vi "Remove Comments.vi"(8 "error in (no error)":errorcluster, 11 "input string":string="{\n\"Cluster\": {\n\"Name\": \"test\", //Represents the name of a person\n\"Department\": \"test2\"/*Gives the department name and \nthe functionality of the department*/\n}") -> (0 "error out":errorcluster, 3 "output String":string)   [LabVIEW 2015]
doc: "This VI removes comments from the JSON that has just been read from a JSON file.This step is mandatory before parsing out the data to the next step. \nIt is capable of removing <b>single line ( // // ) </b>and<b> multiple line (/* */)</b>comments from the input JSON String."
panel:
  # "The input can be changed to test the working of the SubVI"
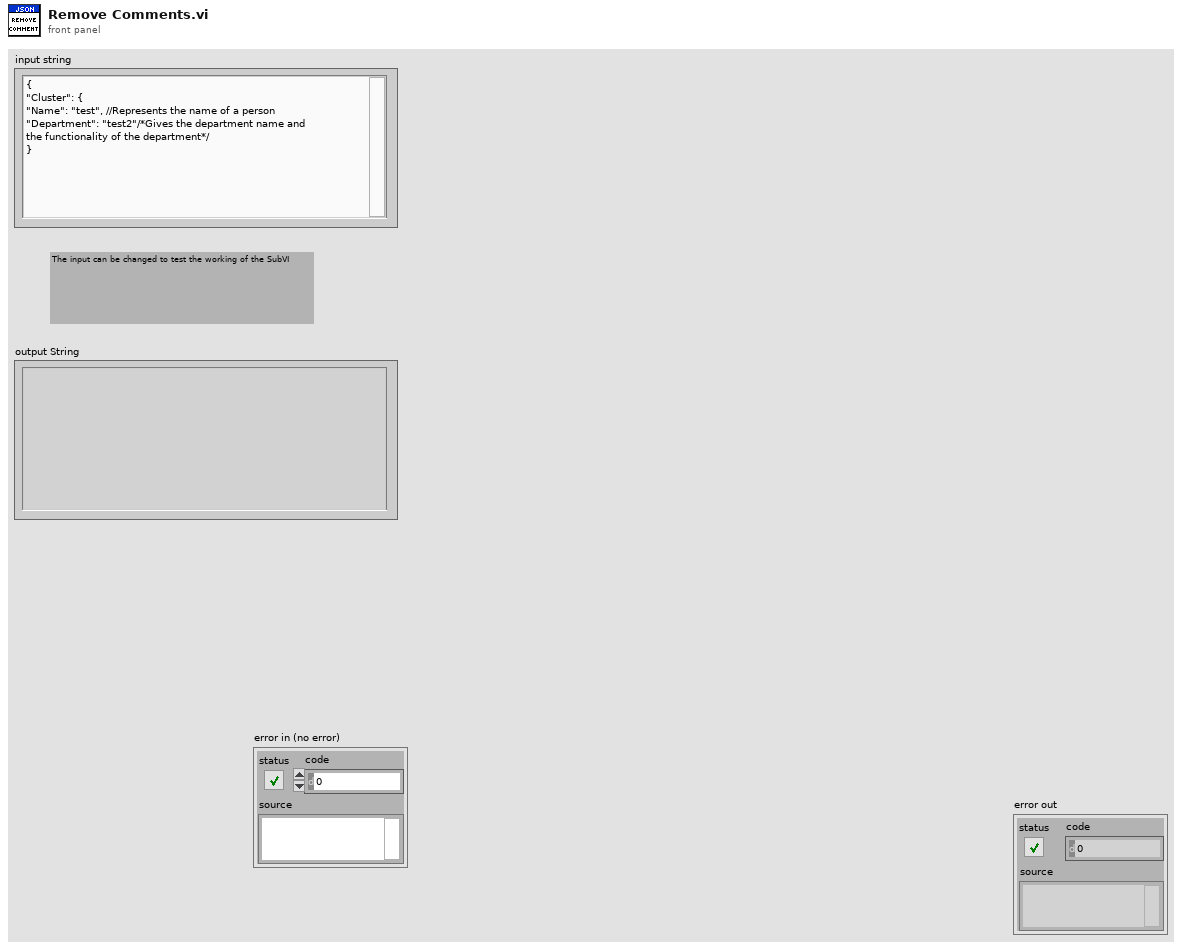
[diagram p1: front panel]
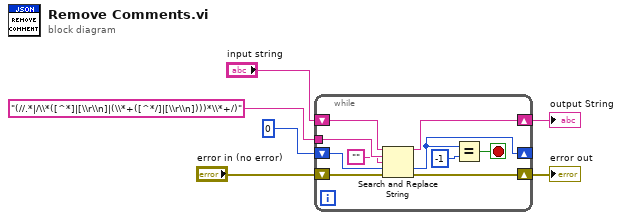
[diagram p0: block diagram]
diagram:
  n1 = while {
    tunnel: "(//.*|/\\*([^*]|[\\r\\n]|(\\*+([^*/]|[\\r\\n])))*\\*+/)" ("regular expression") -> [w16]
    shift-right: [w10] -> w4
    shift-left: "error in (no error)" -> [w11]
    shift-right: [w7] -> _
    shift-left: 0 ("offset past match") -> [w13]
    shift-right: [w14] -> w2
    shift-left: "input string" -> [w12]
    stop <- w8 stop-if-true
    n2 = Search and Replace String(input string=w12, search string=w16, replace string="", offset=w13, error in=w11) -> (result string=w14:string, offset past replacement=w7:i32, error out=w10:errorcluster)  [unwired: 3 in, 1 out]
    n3 = Equal?(x=w7, y=-1) -> (x = y?=w8:bool)
  }
  "error out" <- w4
  "output String" <- w2
